vi "Read Vrange.vi"(8 "error in (no error)":errorcluster, 11 "Set f0 MSG in":refnum<class "Set Vrange MSG.lvclass">) -> (0 "error out":errorcluster, 2 "Vrange":sgl[](array[numeric]), 3 "Set f0 MSG out":refnum<class "Set Vrange MSG.lvclass">)   [LabVIEW 2014, in "ePAS Library.lvlib" / "Set Vrange MSG.lvclass"]
uses:
  Set Vrange MSG.lvclass
  Set Vrange MSG.lvclass/Set Vrange MSG.ctl
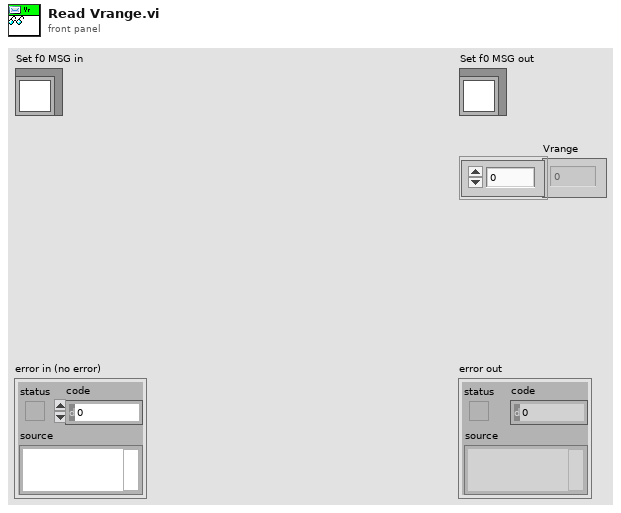
[diagram p1: front panel]
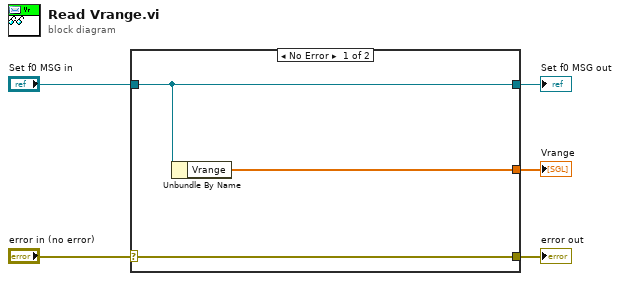
[diagram p0: block diagram]
diagram:
  n1 = case shown="No Error" "error in (no error)" {
    selector: "error in (no error)" -> [w8 w9]
    tunnel: [w8 w9] -> w4
    tunnel: [w7 w10] -> w2
    tunnel: "Set f0 MSG in" -> [w7 w10]
    tunnel: [w6 _] -> w1
    frame No Error {
      n2 = Unbundle By Name(w7) -> ("Vrange"=w6:sgl[])
    }
    frame Error {
    }
  }
  "error out" <- w4
  "Set f0 MSG out" <- w2
  "Vrange" <- w1
